vi "solar_excel Worksheet Read (Sheet).vi"(6 "Truncate Empty Cells? (F)":bool, 8 "error in (no error)":errorcluster, 11 "Excel Worksheet in":T1) -> (0 "error out":errorcluster, 2 "Cells":string[][](array[string]), 3 "Excel Worksheet out":T1)   [LabVIEW 2018]
doc: "This returns all cells from a Worksheet."
uses:
  solar_excel_ctl Worksheet.ctl
  solar_excel_ctl TSV.ctl
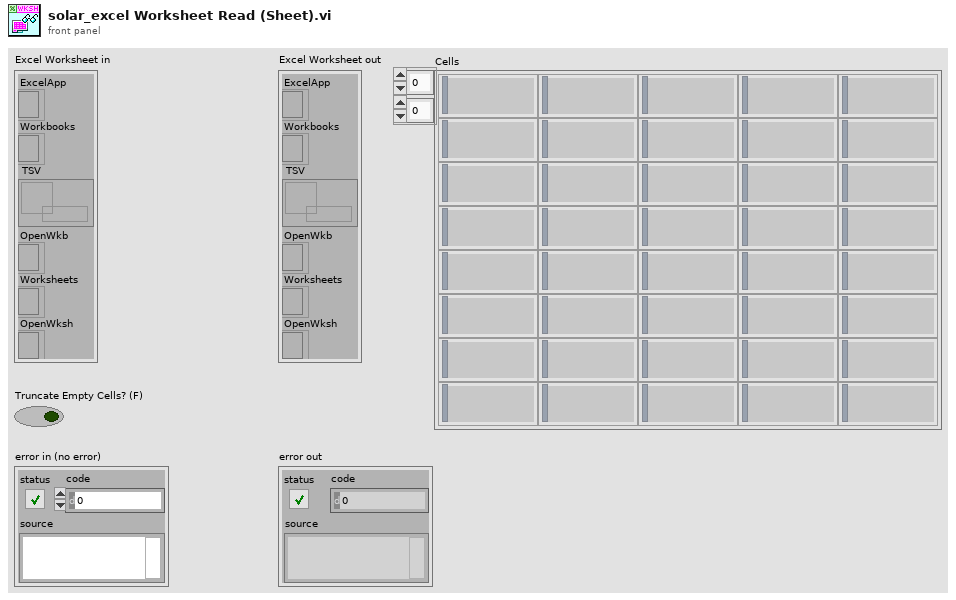
[diagram p1: front panel]
types:
  T1 = typedef "solar_excel_ctl Worksheet.ctl" = cluster{"ExcelApp":refnum<k7>, "Workbooks":refnum<k7>, "TSV":refnum<queue>, "OpenWkb":refnum<k7>, "Worksheets":refnum<k7>, "OpenWksh":refnum<k7>}
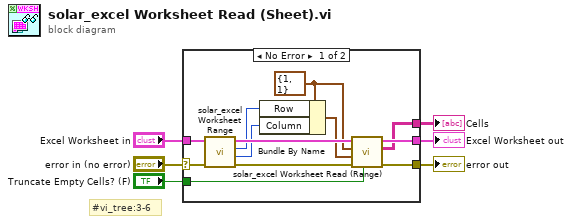
[diagram p0: block diagram]
diagram:
  # "#vi_tree:3-6"
  n1 = case shown="No Error" "error in (no error)" {
    selector: "error in (no error)" -> [w18 w20]
    tunnel: [w9 w20] -> w6
    tunnel: "Excel Worksheet in" -> [w17 w19]
    tunnel: [w10 w19] -> w3
    tunnel: [w8 _] -> w2
    tunnel: "Truncate Empty Cells? (F)" -> [w7 _]
    frame No Error {
      w14 = cluster{"Row":u32, "Column":u32} {"Row"=1, "Column"=1} ("Start (1,1 = 'A1')")
      n2 = call "solar_excel Worksheet Range.vi"("error in (no error)"=w18, "Excel Worksheet in"=w17) -> ("error out"=w16:errorcluster, "Columns"=w12:u32, "Rows"=w13:u32, "Excel Worksheet out"=w15:T1)  [unwired: 6 in]
      n3 = Bundle By Name(cluster=w14, "Row"=w13, "Column"=w12) -> (w11:cluster{"Row":u32, "Column":u32})
      n4 = call "solar_excel Worksheet Read (Range).vi"("Truncate Empty Cells? (F)"=w7, "error in (no error)"=w16, "End (1,1 = 'A1')"=w11, "Start (1,1 = 'A1')"=w14, "Excel Worksheet in"=w15) -> ("error out"=w9:errorcluster, "Cells"=w8:string[][], "Excel Worksheet out"=w10:T1)  [unwired: 4 in]
    }
    frame Error {
    }
  }
  "error out" <- w6
  "Excel Worksheet out" <- w3
  "Cells" <- w2
